vi "Init Sequencing.vi"(8 "error in (no error)":errorcluster, 11 "DaqControl in":refnum<class "DaqControl.lvclass">) -> (0 "error out":errorcluster, 3 "DaqControl out":refnum<class "DaqControl.lvclass">)   [LabVIEW 2020, in "VolatusDaq.lvlib" / "DaqControl.lvclass"]
uses:
  DaqControl.lvclass
  DaqControl.lvclass/DaqControl.ctl
  Seq Cmd Type.ctl
  Seq Cmd.ctl
  Seq Action Type.ctl
  VolatusDaq.lvlib
  Sequence Action.ctl
  Sequencing Qs.ctl
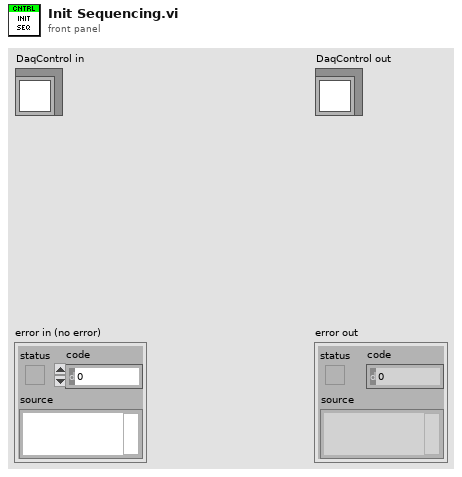
[diagram p1: front panel]
types:
  T1 = typedef "VolatusDaq.lvlib/DaqControl.lvclass/Sequencing Qs.ctl" = cluster{"Seqs":refnum<queue>[], "Aborts":refnum<queue>[]}
  T2 = typedef "VolatusDaq.lvlib/DaqControl.lvclass/Seq Cmd.ctl" = cluster{"Type":T3, "Seq Index":i32}
  T3 = typedef "VolatusDaq.lvlib/DaqControl.lvclass/Seq Cmd Type.ctl" = enum16{"Timeout", "Abort", "Reset Ticks", "Prepare", "Start"}
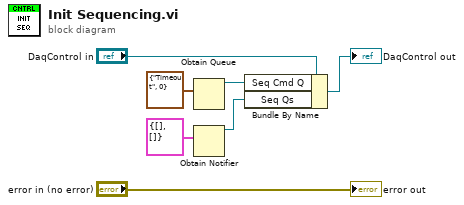
[diagram p0: block diagram]
diagram:
  n1 = Obtain Queue(element data type=T2 {"Type"=enum."Timeout", "Seq Index"=0} ("Seq Cmd")) -> (queue out=w3:refnum<queue>)  [unwired: 4 in, 2 out]
  n2 = Obtain Notifier(notification data type=T1 {"Seqs"=[], "Aborts"=[]} ("Sequencing Qs")) -> (notifier out=w1:refnum<notifier>)  [unwired: 3 in, 2 out]
  n3 = Bundle By Name(cluster="DaqControl in", "Seq Cmd Q"=w3, "Seq Qs"=w1) -> (→"DaqControl out":refnum<class "DaqControl.lvclass">)
  "error out" <- "error in (no error)"
